vi "02_CMD_loop.vi"(11 "VISA resource name":refnum<visa-resource-name>) -> ()   [LabVIEW 2017]
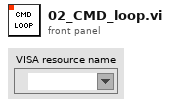
[diagram p1: front panel]
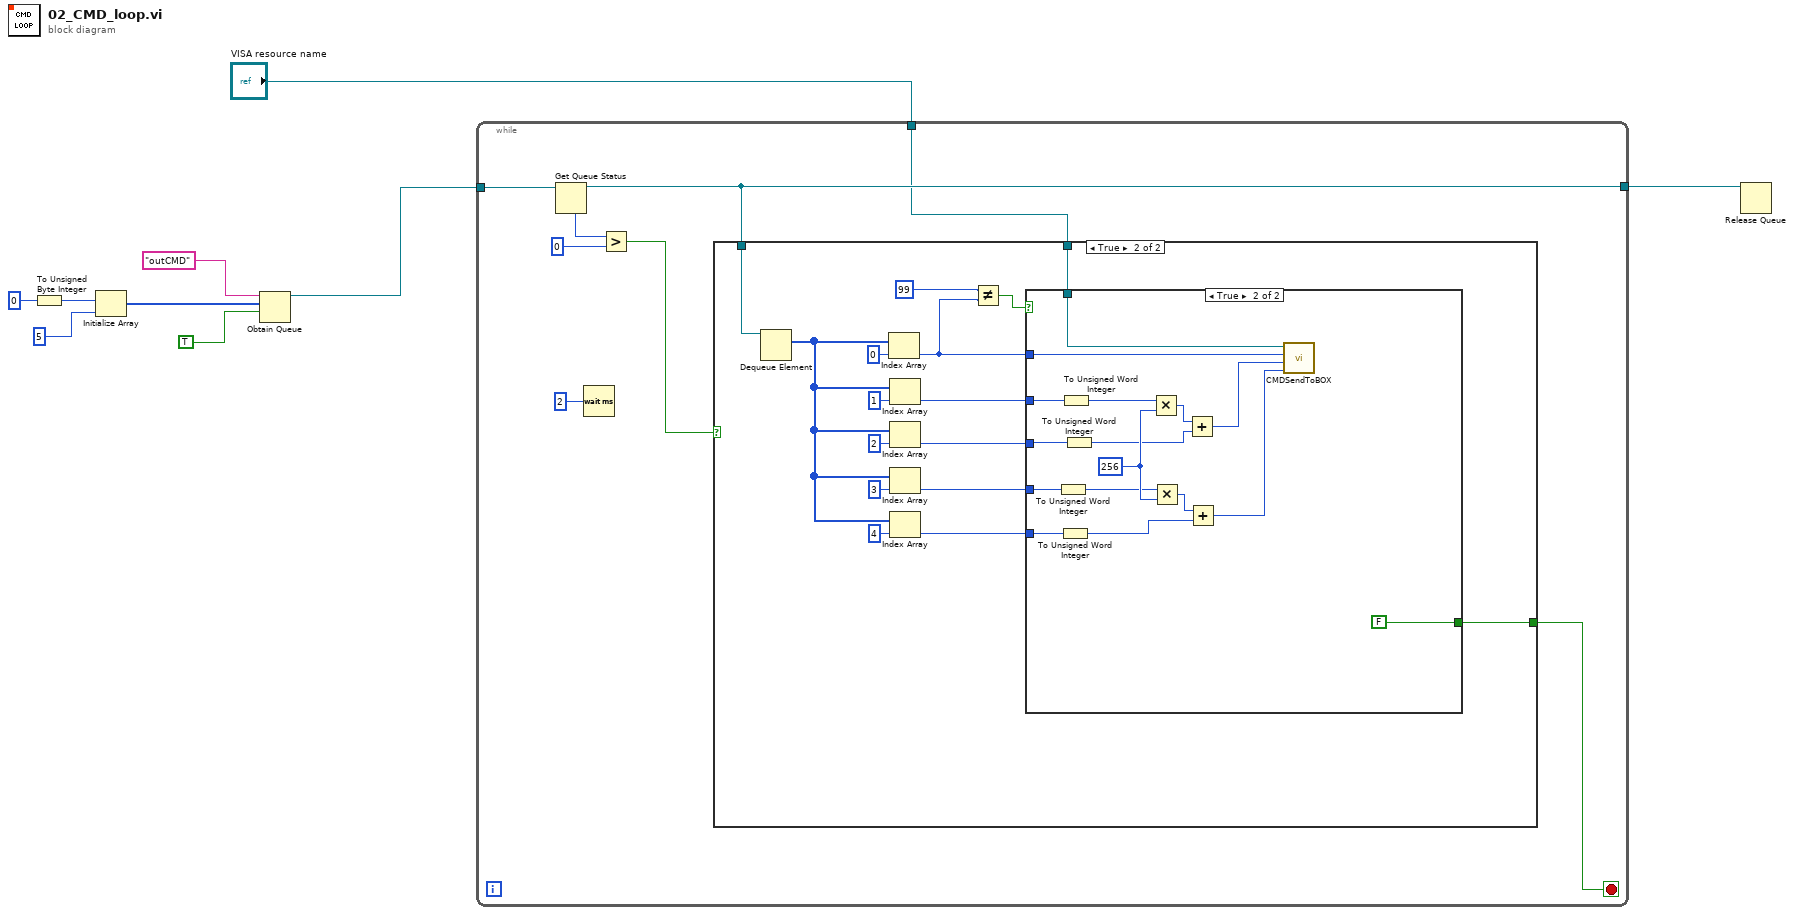
[diagram p0: block diagram]
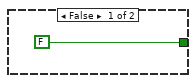
[diagram p2: hidden frame]
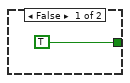
[diagram p3: hidden frame]
diagram:
  n1 = To Unsigned Byte Integer(number=u8 0) -> (unsigned 8bit integer=w7:u8)
  n2 = Initialize Array(w7, 5 ("dimension size")) -> (w4:u8[])
  n3 = Obtain Queue(name (unnamed)="outCMD", element data type=w4, create if not found? (T)=TRUE) -> (queue out=w2:refnum<queue>)  [unwired: 2 in, 2 out]
  n4 = while {
    tunnel: w2 -> [w17]
    tunnel: [w13] -> w9
    tunnel: "VISA resource name" -> [w12]
    stop <- w11 stop-if-true
    n5 = Get Queue Status(queue=w17) -> (queue out=w13:refnum<queue>, # elements in queue=w16:i32)  [unwired: 2 in, 6 out]
    n6 = Wait (ms)(milliseconds to wait=u32 2) -> ()  [unwired: 1 out]
    n7 = Greater?(x=w16, y=0) -> (0:w14:bool)
    n8 = case shown="True" w14 {
      tunnel: w13 -> [_ w34]
      tunnel: w12 -> [_ w23]
      tunnel: [FALSE w22] -> w11
      frame False {
      }
      frame True {
        n9 = Dequeue Element(queue=w34) -> (element=w33:u8[])  [unwired: 2 in, 3 out]
        n10 = Index Array(array=w33, index=0) -> (element=w20:u8)
        n11 = Index Array(array=w33, index=1) -> (element=w27:u8)
        n12 = Index Array(array=w33, index=2) -> (element=w26:u8)
        n13 = Index Array(array=w33, index=3) -> (element=w25:u8)
        n14 = Index Array(array=w33, index=4) -> (element=w24:u8)
        n15 = Not Equal?(x=u8 99, y=w20) -> (x != y?=w19:bool)
        n16 = case shown="True" w19 {
          tunnel: w20 -> [_ w46]
          tunnel: w27 -> [_ w42]
          tunnel: w26 -> [_ w40]
          tunnel: w25 -> [_ w38]
          tunnel: w24 -> [_ w36]
          tunnel: w23 -> [_ w45]
          tunnel: [TRUE FALSE] -> w22
          frame False {
          }
          frame True {
            w47 = i16 256 ("y")
            n17 = To Unsigned Word Integer(number=w38) -> (unsigned 16bit integer=w39:u16)
            n18 = To Unsigned Word Integer(number=w36) -> (unsigned 16bit integer=w37:u16)
            n19 = To Unsigned Word Integer(number=w42) -> (unsigned 16bit integer=w43:u16)
            n20 = To Unsigned Word Integer(number=w40) -> (unsigned 16bit integer=w41:u16)
            n21 = Multiply(x=w43, y=w47) -> (x*y=w51:u16)
            n22 = Multiply(x=w39, y=w47) -> (x*y=w50:u16)
            n23 = Add(x=w51, y=w41) -> (x+y=w49:u16)
            n24 = Add(x=w50, y=w37) -> (x+y=w48:u16)
            n25 = call "CMDSendToBOX.vi"("arg2"=w48, "arg1"=w49, "CMD"=w46, "VISA resource name"=w45) -> ()  [unwired: 7 in, 1 out]
          }
        }
      }
    }
  }
  n26 = Release Queue(queue=w9) -> ()  [unwired: 2 in, 3 out]
